vi "test_libssh2_session_init_ex (recv callback).vi"() -> ()   [LabVIEW 2017, in "integration_tests.lvlib"]
uses:
  integration_tests.lvlib
  libssh2/libssh2_session_abstract.ctl
  libssh2/libssh2_session_callback_type.ctl
  libssh2/libssh2_session_handshake_tcp.vi
  libssh2/libssh2_init_default.vi
  <vilib>/Utility/tcp.llb/TCP Get Raw Net Object.vi
  libssh2/libssh2_session_handshake_socket.vi
  libssh2/libssh2_session_disconnect_ex.vi
  libssh2/libssh2.lvlib
  support/support.lvlib
  <vilib>/PNR/Transparent Assertions/Transparent Assertions/Transparent Assertions.lvlib
panel:
  out "error out":errorcluster
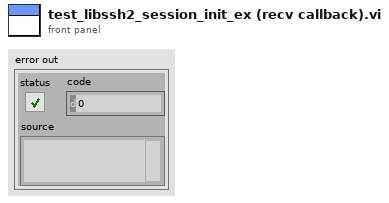
[diagram p1: front panel]
types:
  T1 = typedef "libssh2.lvlib/libssh2_session_abstract.ctl" = cluster{"send":refnum<vi>, "receive":refnum<vi>, "keyboard-interactive response":refnum<vi>}
  T2 = typedef "libssh2.lvlib/libssh2_session_callback_type.ctl" = enum16{"Ignore", "Debug", "Disconnect", "MAC Error", "X11", "Send", "Receive", "Auth Agent", "Auth Agent Identities", "Auth Agent Sign"}
  T3 = typedef "libssh2.lvlib/Session Refnum.ctl" = refnum<k1>
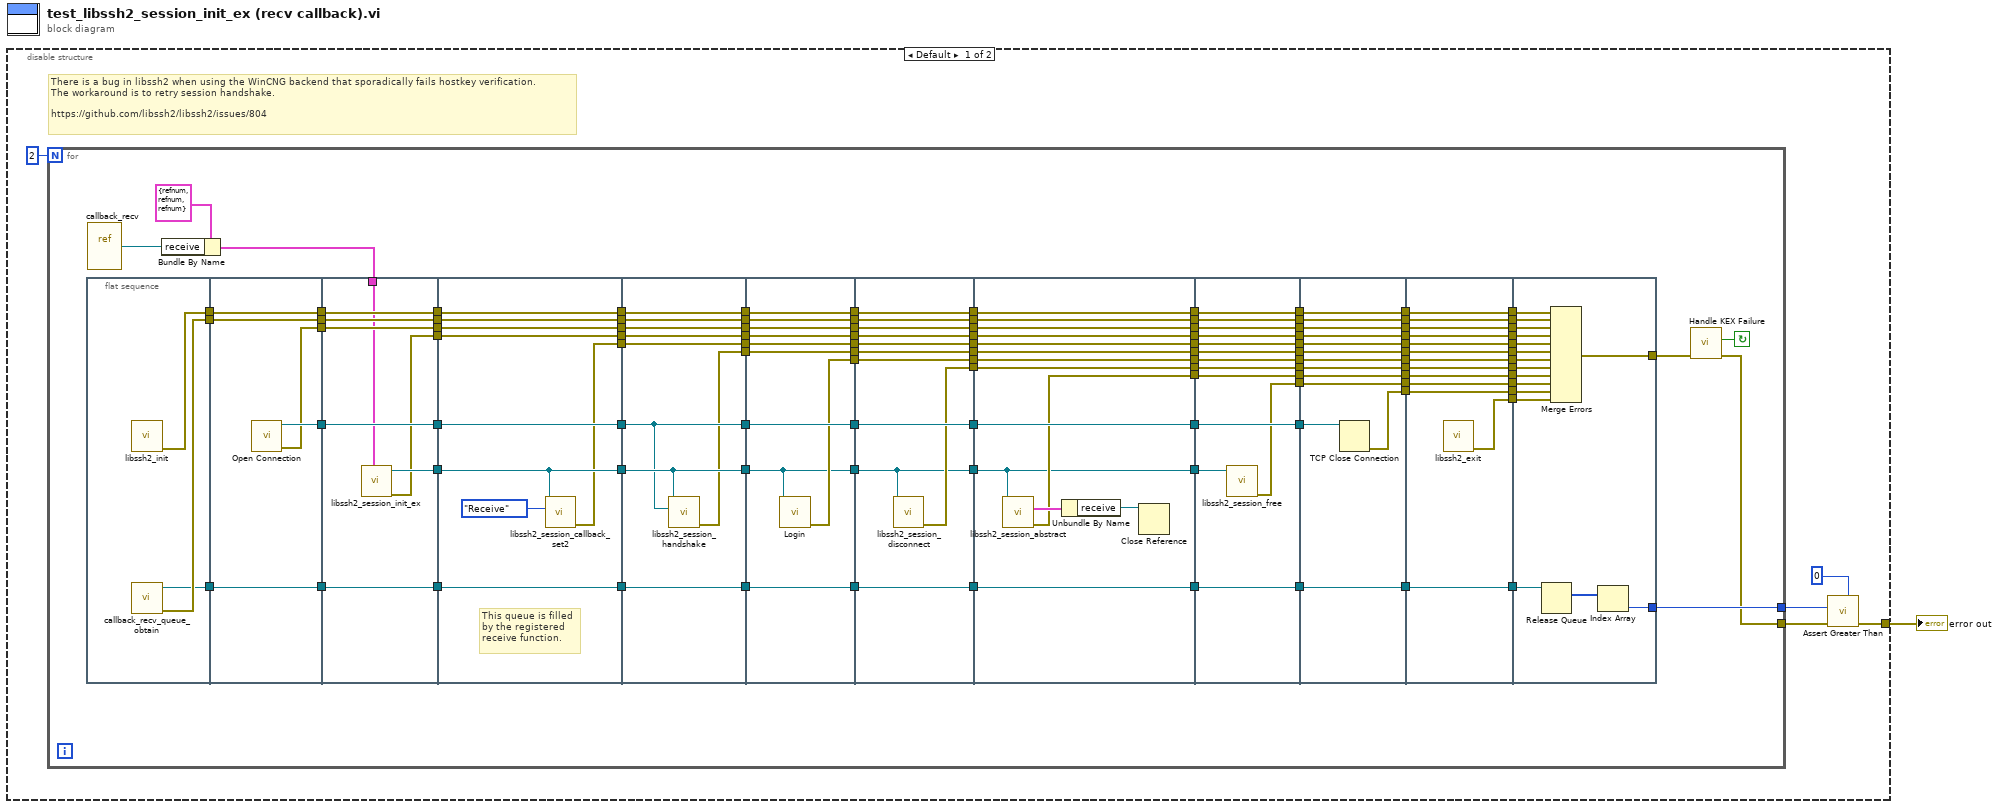
[diagram p0: block diagram]
diagram:
  n1 = disable-structure "Diagram Disable Structure" shown="Default" {
    disable-tunnel: [w6 _] -> w1
    frame condition #0 (active) {
      # "There is a bug in libssh2 when using the WinCNG backend that sporadically fails hostkey verification.\nThe workaround is to retry session handshake.\n\nhttps://github.com/libssh2/libssh2/issues/804"
      n2 = for {
        N: 2 -> [_]
        tunnel: [w10] -> w3
        tunnel: [w7] -> w5
        stop <- w8 continue-if-true
        n3 = flat-sequence {
          tunnel: [w118] -> w115
          tunnel: [w117] -> w114
          tunnel: [w116] -> w113
          tunnel: [w123] -> w112
          tunnel: w115 -> [w122]
          tunnel: [w122] -> w111
          tunnel: [w121] -> w110
          tunnel: w114 -> [w120]
          tunnel: [w120] -> w109
          tunnel: [w119] -> w108
          tunnel: w113 -> [w119]
          tunnel: w112 -> [w131]
          tunnel: [w131] -> w107
          tunnel: w111 -> [w130]
          tunnel: [w130] -> w106
          tunnel: w110 -> [w129]
          tunnel: [w129] -> w105
          tunnel: [w128] -> w104
          tunnel: [w127] -> w103
          tunnel: w109 -> [w126]
          tunnel: [w126] -> w102
          tunnel: w11 -> [w125]
          tunnel: [w124] -> w101
          tunnel: w108 -> [w124]
          tunnel: w107 -> [w140]
          tunnel: [w140] -> w100
          tunnel: w106 -> [w139]
          tunnel: [w139] -> w99
          tunnel: w105 -> [w138]
          tunnel: [w138] -> w98
          tunnel: w104 -> [w134]
          tunnel: [w134] -> w97
          tunnel: w103 -> [w137]
          tunnel: [w137] -> w96
          tunnel: w102 -> [w136]
          tunnel: [w136] -> w95
          tunnel: [w133] -> w94
          tunnel: [w132] -> w93
          tunnel: w101 -> [w132]
          tunnel: w100 -> [w145]
          tunnel: [w145] -> w92
          tunnel: w99 -> [w149]
          tunnel: [w149] -> w91
          tunnel: w98 -> [w148]
          tunnel: [w148] -> w90
          tunnel: [w147] -> w89
          tunnel: w97 -> [w147]
          tunnel: w96 -> [w146]
          tunnel: [w146] -> w88
          tunnel: [w144] -> w87
          tunnel: w95 -> [w143]
          tunnel: [w143] -> w86
          tunnel: w94 -> [w142]
          tunnel: [w142] -> w85
          tunnel: [w141] -> w84
          tunnel: w93 -> [w141]
          tunnel: w92 -> [w159]
          tunnel: [w159] -> w83
          tunnel: w91 -> [w158]
          tunnel: [w158] -> w82
          tunnel: w90 -> [w157]
          tunnel: [w157] -> w81
          tunnel: w89 -> [w151]
          tunnel: w88 -> [w156]
          tunnel: [w156] -> w80
          tunnel: w87 -> [w155]
          tunnel: [w155] -> w79
          tunnel: w86 -> [w154]
          tunnel: [w154] -> w78
          tunnel: w85 -> [w153]
          tunnel: [w153] -> w77
          tunnel: [w152] -> w76
          tunnel: [w151] -> w75
          tunnel: [w150] -> w74
          tunnel: w84 -> [w150]
          tunnel: w83 -> [w170]
          tunnel: [w170] -> w73
          tunnel: w82 -> [w169]
          tunnel: [w169] -> w72
          tunnel: w81 -> [w168]
          tunnel: [w168] -> w71
          tunnel: w80 -> [w167]
          tunnel: [w167] -> w70
          tunnel: [w166] -> w69
          tunnel: w79 -> [w165]
          tunnel: [w165] -> w68
          tunnel: w78 -> [w164]
          tunnel: [w164] -> w67
          tunnel: w77 -> [w163]
          tunnel: [w163] -> w66
          tunnel: w76 -> [w162]
          tunnel: [w162] -> w65
          tunnel: [w161] -> w64
          tunnel: w75 -> [w161]
          tunnel: [w160] -> w63
          tunnel: w74 -> [w160]
          tunnel: w73 -> [w184]
          tunnel: [w184] -> w62
          tunnel: w72 -> [w183]
          tunnel: [w183] -> w61
          tunnel: w71 -> [w182]
          tunnel: [w182] -> w60
          tunnel: w70 -> [w181]
          tunnel: [w181] -> w59
          tunnel: w69 -> [w180]
          tunnel: [w180] -> w58
          tunnel: w68 -> [w179]
          tunnel: [w179] -> w57
          tunnel: w67 -> [w178]
          tunnel: [w178] -> w56
          tunnel: w66 -> [w177]
          tunnel: [w177] -> w55
          tunnel: w65 -> [w176]
          tunnel: [w176] -> w54
          tunnel: w64 -> [w172]
          tunnel: [w173] -> w53
          tunnel: [w172] -> w52
          tunnel: [w171] -> w51
          tunnel: w63 -> [w171]
          tunnel: w62 -> [w197]
          tunnel: [w197] -> w50
          tunnel: w61 -> [w196]
          tunnel: [w196] -> w49
          tunnel: w60 -> [w195]
          tunnel: [w195] -> w48
          tunnel: w59 -> [w194]
          tunnel: [w194] -> w47
          tunnel: w58 -> [w193]
          tunnel: [w193] -> w46
          tunnel: w57 -> [w192]
          tunnel: [w192] -> w45
          tunnel: w56 -> [w191]
          tunnel: [w191] -> w44
          tunnel: w55 -> [w190]
          tunnel: [w190] -> w43
          tunnel: w54 -> [w189]
          tunnel: [w189] -> w42
          tunnel: w53 -> [w188]
          tunnel: [w188] -> w41
          tunnel: w52 -> [w187]
          tunnel: [w186] -> w40
          tunnel: [w185] -> w39
          tunnel: w51 -> [w185]
          tunnel: w50 -> [w210]
          tunnel: w49 -> [w209]
          tunnel: [w209] -> w38
          tunnel: w48 -> [w208]
          tunnel: [w208] -> w37
          tunnel: [w207] -> w36
          tunnel: w47 -> [w206]
          tunnel: [w206] -> w35
          tunnel: w46 -> [w205]
          tunnel: [w205] -> w34
          tunnel: w45 -> [w204]
          tunnel: [w204] -> w33
          tunnel: w44 -> [w203]
          tunnel: [w203] -> w32
          tunnel: w43 -> [w202]
          tunnel: [w202] -> w31
          tunnel: w42 -> [w201]
          tunnel: [w201] -> w30
          tunnel: w41 -> [w200]
          tunnel: [w200] -> w29
          tunnel: [w199] -> w28
          tunnel: w40 -> [w199]
          tunnel: [w198] -> w27
          tunnel: w39 -> [w198]
          tunnel: w38 -> [w223]
          tunnel: [w223] -> w26
          tunnel: w37 -> [w222]
          tunnel: [w222] -> w25
          tunnel: w36 -> [w221]
          tunnel: [w221] -> w24
          tunnel: [w220] -> w23
          tunnel: w35 -> [w219]
          tunnel: [w219] -> w22
          tunnel: w34 -> [w218]
          tunnel: [w218] -> w21
          tunnel: w33 -> [w217]
          tunnel: [w217] -> w20
          tunnel: w32 -> [w216]
          tunnel: [w216] -> w19
          tunnel: w31 -> [w215]
          tunnel: [w215] -> w18
          tunnel: w30 -> [w214]
          tunnel: [w214] -> w17
          tunnel: w29 -> [w213]
          tunnel: [w213] -> w16
          tunnel: [w212] -> w15
          tunnel: w28 -> [w212]
          tunnel: [w211] -> w14
          tunnel: w27 -> [w211]
          tunnel: w26 -> [w239]
          tunnel: w25 -> [w238]
          tunnel: w24 -> [w237]
          tunnel: w23 -> [w236]
          tunnel: w22 -> [w235]
          tunnel: w21 -> [w234]
          tunnel: w20 -> [w233]
          tunnel: w19 -> [w232]
          tunnel: w18 -> [w231]
          tunnel: w17 -> [w230]
          tunnel: w16 -> [w229]
          tunnel: w15 -> [w228]
          tunnel: w14 -> [w226]
          tunnel: [w225] -> w9
          tunnel: [w224] -> w10
          frame #0 {
            n4 = call-poly "libssh2_init.vi"() -> ("error out"=w118:errorcluster)  [unwired: 11 in]
            n5 = call "callback_recv_queue_obtain.vi"() -> ("error out"=w117:errorcluster, "queue out"=w116:refnum<queue>)  [unwired: 10 in]
          }
          frame #1 {
            n6 = call "Open Connection.vi"() -> ("error out"=w121:errorcluster, "connection ID"=w123:refnum<k5>)  [unwired: 10 in]
          }
          frame #2 {
            n7 = call "libssh2_session_init_ex.vi"("abstract"=w125) -> ("error out"=w127:errorcluster, "session"=w128:T3)  [unwired: 9 in]
          }
          frame #3 {
            # "This queue is filled\nby the registered\nreceive function."
            n8 = call "libssh2_session_callback_set2.vi"("callback type"=libssh2_session_callback_type."Receive", "session"=w134) -> ("error out"=w133:errorcluster)  [unwired: 8 in, 1 out]
          }
          frame #4 {
            n9 = call-poly "libssh2_session_handshake.vi"("tcp connection"=w145, "session"=w147) -> ("error out"=w144:errorcluster)  [unwired: 9 in]
          }
          frame #5 {
            n10 = call "Login.vi"("session"=w151) -> ("error out"=w152:errorcluster)  [unwired: 10 in]
          }
          frame #6 {
            n11 = call "libssh2_session_disconnect.vi"("session"=w161) -> ("error out"=w166:errorcluster)  [unwired: 10 in]
          }
          frame #7 {
            n12 = call "libssh2_session_abstract.vi"("session"=w172) -> ("error out"=w173:errorcluster, "abstract"=w175:T1)  [unwired: 9 in]
            n13 = Unbundle By Name(w175) -> ("receive"=w174:refnum<vi>)
            n14 = Close Reference(reference=w174) -> ()  [unwired: 1 in, 1 out]
          }
          frame #8 {
            n15 = call "libssh2_session_free.vi"("session"=w187) -> ("error out"=w186:errorcluster)  [unwired: 10 in]
          }
          frame #9 {
            n16 = TCP Close Connection(connection ID=w210) -> (error out=w207:errorcluster)  [unwired: 2 in, 1 out]
          }
          frame #10 {
            n17 = call "libssh2_exit.vi"() -> ("error out"=w220:errorcluster)  [unwired: 11 in]
          }
          frame #11 {
            n18 = Release Queue(queue=w226) -> (remaining elements=w227:i32[])  [unwired: 2 in, 2 out]
            n19 = Merge Errors(w239, w232, w238, w235, w231, w233, w230, w234, w229, w228, w237, w236) -> (w225:errorcluster)
            n20 = Index Array(array=w227) -> (element=w224:i32)  [unwired: 1 in]
          }
        }
        n21 = vi-ref "callback_recv.vi"() -> (w12:refnum<vi>)
        n22 = Bundle By Name(cluster=T1 {"send"=refnum, "receive"=refnum, "keyboard-interactive response"=refnum} ("abstract"), "receive"=w12) -> (w11:T1)
        n23 = call "Handle KEX Failure.vi"("error in (no error)"=w9) -> ("error out"=w7:errorcluster, "KEX Failure"=w8:bool)  [unwired: 9 in]
      }
      n24 = call <vilib>:"Assert Greater Than.vi"("Expected"=i64 0, "error in (no error)"=w5, "Actual"=w3) -> ("error out"=w6:errorcluster)  [unwired: 8 in]
    }
    frame condition #1 {
    }
  }
  "error out" <- w1
